vi "Get Keyboard Information.vi"(8 "error in (no error)":errorcluster) -> (0 "error out":errorcluster, 3 "HKL":u64)   [LabVIEW 2020, in "MacroAssert.lvlib" / "Win Util.lvlib"]
uses:
  Win Util.lvlib
  user32.dll
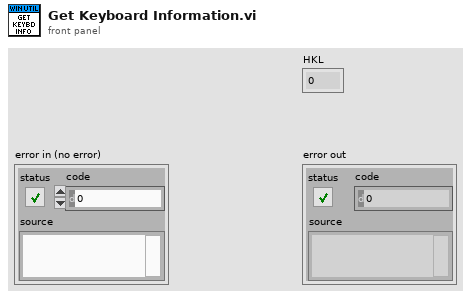
[diagram p1: front panel]
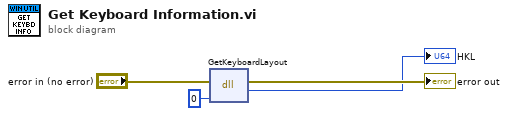
[diagram p0: block diagram]
diagram:
  n1 = dll-call lib="user32.dll" fn="GetKeyboardLayout"(error in="error in (no error)", "idThread"=u32 0) -> (error out=→"error out":errorcluster, "HKL"=→"HKL":u64)  [unwired: 3 in, 1 out]
